vi "Do Request.vi"(7 "Processing In":refnum<class "Processing.lvclass">, 11 "Scores in":refnum<class "Scores.lvclass">) -> (0 "error out":errorcluster, 5 "Processing":refnum<class "Processing.lvclass">)   [LabVIEW 2020, in "Scores.lvclass"]
uses:
  Scores.lvclass
  Scores.lvclass/Scores.ctl
  <vilib>/IlluminatedG/IG HTTP Server/HTTP Server/Processing/Processing.lvclass
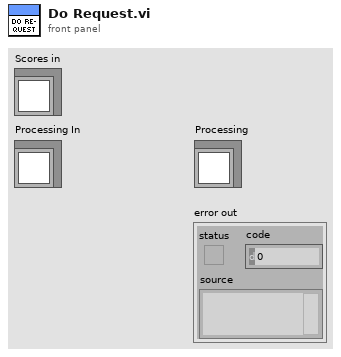
[diagram p1: front panel]
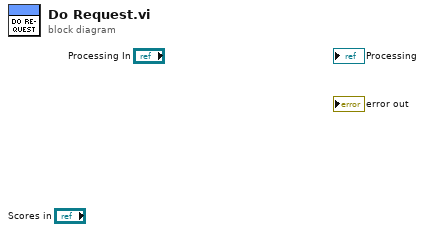
[diagram p0: block diagram]
diagram:
